vi "DeleteFile.vi"(0 "Item Refnum":refnum<vi>, 11 "error in":errorcluster) -> (15 "error out":errorcluster)   [LabVIEW 2020]
doc: "Deletes a project item from the project and deletes the item from disk\n\nCreated by Bas v. Etten 2023"
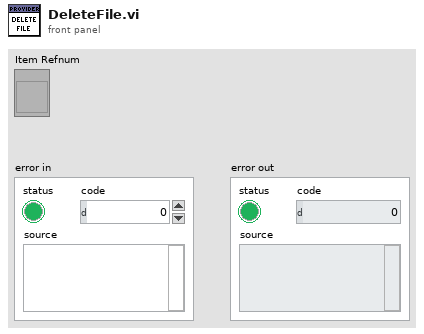
[diagram p1: front panel]
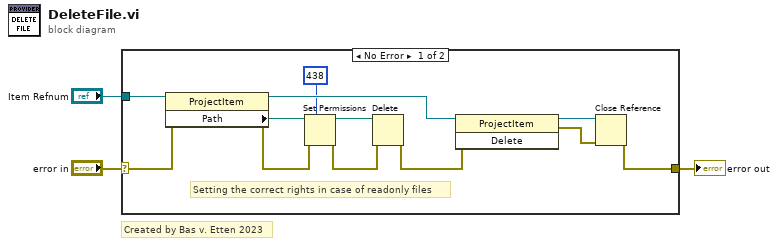
[diagram p0: block diagram]
diagram:
  # "Created by Bas v. Etten 2023"
  n1 = case shown="No Error" "error in" {
    selector: "error in" -> [w9 w16]
    tunnel: [w15 w16] -> w2
    tunnel: "Item Refnum" -> [w11 _]
    frame No Error {
      # "Setting the correct rights in case of readonly files"
      n2 = property class="ProjectItem"(reference=w11, error in=w9) -> (reference out=w10:refnum<vi>, error out=w5:errorcluster, "Path"=w7:path)
      n3 = Set Permissions(7:i16 438 ("permissions"), 8:w5, 11:w7) -> (0:w4:errorcluster, 3:w6:path)  [unwired: 2 in]
      n4 = Delete(path (use dialog)=w6, error in=w4) -> (error out=w14:errorcluster)  [unwired: 3 in, 2 out]
      n5 = invoke class="ProjectItem" method="Delete"(reference=w10, error in=w14) -> (reference out=w13:refnum<vi>, error out=w12:errorcluster)  [unwired: 1 in, 1 out]
      n6 = Close Reference(reference=w13, error in (no error)=w12) -> (error out=w15:errorcluster)
    }
    frame Error {
    }
  }
  "error out" <- w2
